vi "Update Zoom.vi"(8 "error in (no error)":errorcluster, 10 "Zoom":bool, 11 "XYGraphOverview in":refnum<class "XYGraphOverview.lvclass">) -> (0 "error out":errorcluster, 3 "XYGraphOverview out":refnum<class "XYGraphOverview.lvclass">)   [LabVIEW 2020, in "XYGraphOverview.lvlib" / "XYGraphOverview.lvclass"]
uses:
  XYGraphOverview.lvclass
  Caller User Event Data.ctl
  Command.ctl
  XYGraphOverview.lvclass/XYGraphOverview.ctl
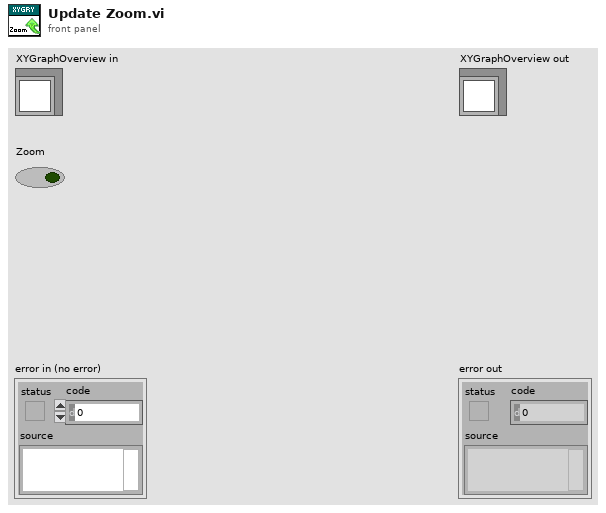
[diagram p1: front panel]
types:
  T1 = typedef "XYGraphOverview.lvlib/XYGraphOverview.lvclass/Caller User Event Data.ctl" = cluster{"Command":T2, "Data":variant}
  T2 = typedef "XYGraphOverview.lvlib/XYGraphOverview.lvclass/Command.ctl" = enum16{"Update Data", "Update Limit", "Zoom"}
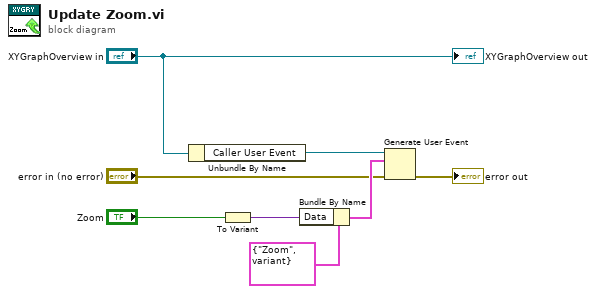
[diagram p0: block diagram]
diagram:
  n1 = Unbundle By Name("XYGraphOverview in") -> ("Caller User Event"=w8:refnum<user-event>)
  n2 = To Variant(anything="Zoom") -> (Variant=w6:variant)
  n3 = Bundle By Name(cluster=T1 {"Command"=enum."Zoom", "Data"=variant} ("event data"), "Data"=w6) -> (w5:T1)
  n4 = Generate User Event(user event=w8, event data cluster=w5, error in="error in (no error)") -> (error out=→"error out":errorcluster)  [unwired: 1 in, 1 out]
  "XYGraphOverview out" <- "XYGraphOverview in"
